vi "Set Equation Para.vi"(8 "error in (no error)":errorcluster, 10 "parameter":variant, 11 "PDE in":refnum<class "NI_PDE.lvclass">) -> (0 "error out":errorcluster, 3 "PDE out":refnum<class "NI_PDE.lvclass">)   [LabVIEW 2017, in "NI_PDE.lvlib" / "NI_PDE.lvclass"]
uses:
  <vilib>/gmath/pde.llb/PDEClass/NI_PDE.lvclass
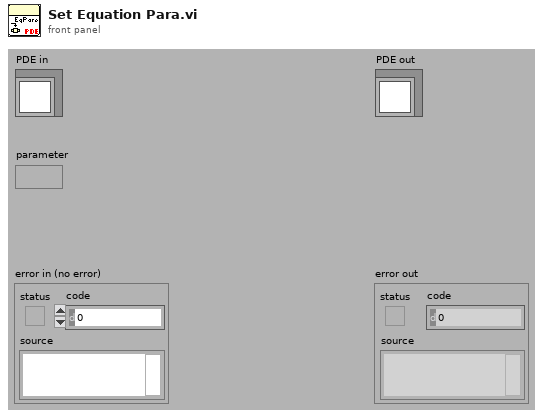
[diagram p1: front panel]
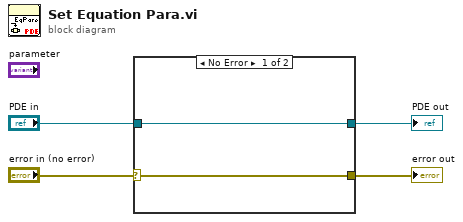
[diagram p0: block diagram]
diagram:
  n1 = case shown="No Error" "error in (no error)" {
    selector: "error in (no error)" -> [w5 w8]
    tunnel: "PDE in" -> [w6 w7]
    tunnel: [w6 w7] -> w3
    tunnel: [w5 w8] -> w2
    frame No Error {
    }
    frame Error {
    }
  }
  "PDE out" <- w3
  "error out" <- w2
